vi "fFPGA Initialization.vi"(4 "Testpulse Cluster":T4={"Master Pulser On/Off"=FALSE, "Testpulse Turnaround Time (samples)"=14, "Pulse Separation (samples)"=0, "Pulse duration (samples)"=0}, 5 "DAQ Info Cluster":T3={"Data Chunks per File"=1000, "Samples per Waveform"=95, "Pretrigger Samples"=15, "circular buffer length (samples)"=1000, "Waveforms per Data Chunk"=5000} {"Waveforms per Data Chunk" format="%.2p"}, 6 "Channel Cluster":T2={"det_type"=[], "Serial numbers"=[], "Sources"=[], "Trigger level"=[4000, 4000, 4000, 4000, 4000, 4000, 4000, 4000], "Data Record On/Off"=[], "Number of Channels"=8}, 7 "General Cluster":cluster{"Location":i16} {"Location" items=["Purdue", "NIKHEF", "Zurich", "???"]}, 8 "error in":errorcluster, 11 "FPGA VI Reference In":T1) -> (0 "error out":errorcluster, 3 "FPGA VI Reference Out":T1)   [LabVIEW 2012]
uses:
  FPGA Bitfiles/ModuFPGAtype.ctl
  <vilib>/FPGAPlugInAG/PXI-7951R/niLvFpga_Reset_PXI-7951R.vi
  <vilib>/Utility/error.llb/Error Cluster From Error Code.vi
  <vilib>/LabVIEW Targets/FPGA/FlexRIO/CustomFPGAMethods/79XXR_Method_IOModuleStatusImpl.vi
  <vilib>/FPGAPlugInAG/PXI-7951R/niLvFpga_Run_PXI-7951R.vi
  <vilib>/rvi/errors/niLvFpgaAdjustHostInterfaceError.vi
  Program Files (x86)/National Instruments/LabVIEW 2012/Targets/NI/FPGA/StockFPGA_IntfPrivate/ScriptTemplates/StockFPGA_PlugInRead32.vi
  <vilib>/rvi/interface/nirviMethod/nirviMethod.xnode
  FPGA Bitfiles/ModuDAQ_FPGATarget_ModuFPGAdark_Chz-m0P+4co.lvbitx
  <vilib>/rvi/interface/nirviReadWriteControl/nirviReadWriteControl.xnode
  <vilib>/rvi/errors/niLvFpgaMergeErrorWithErrorCode.vi
  NiFpgaLv.dll
  <vilib>/FPGAPlugInAG/PXI-7951R/niLvFpga_Read32_PXI-7951R.vi
  <vilib>/rvi/interface/nirviReadWriteControl/niFpgaRWControlAccessTimeoutTemplate.vi
  <vilib>/FPGAPlugInAG/PXI-7951R/niLvFpga_ConfigureFifo_PXI-7951R.vi
  <vilib>/FPGAPlugInAG/PXI-7951R/niLvFpga_StartFifo_PXI-7951R.vi
panel:
  # "Channel 0"
  # "Channel 1"
  # "Channel 2"
  # "Channel 3"
  # "Channel 4"
  # "Channel 5"
  # "Channel 6"
  # "Channel 7"
  # "Waveform/Data Chunk information"
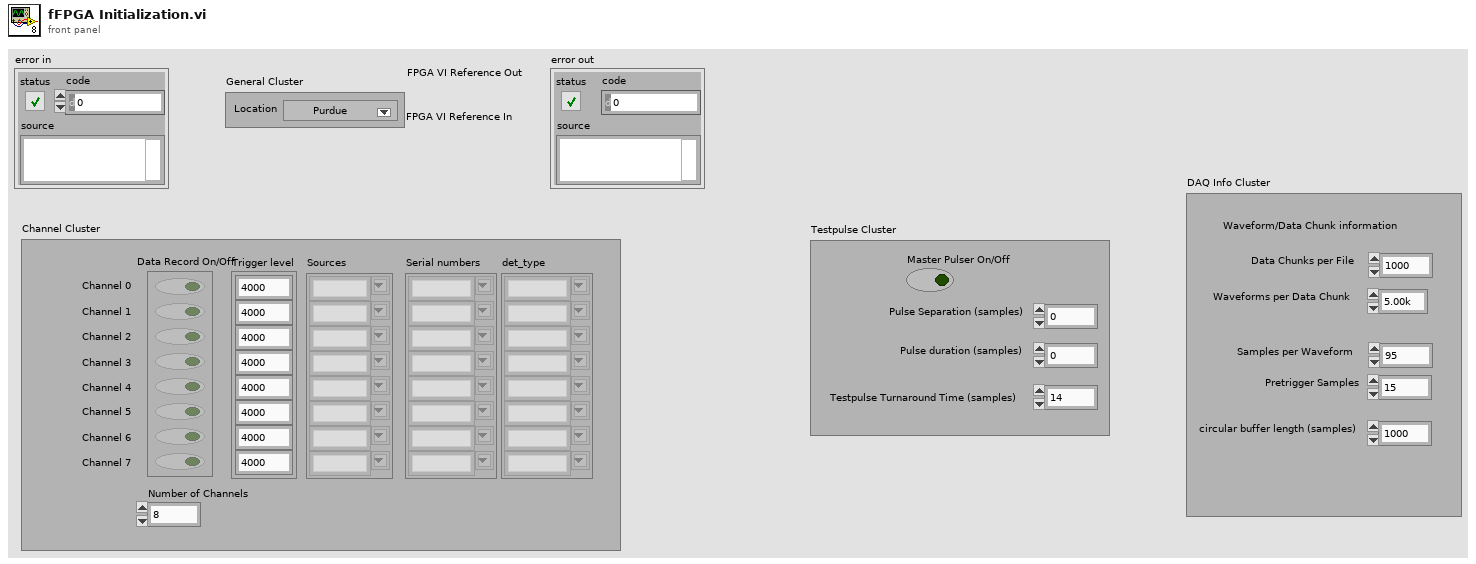
[diagram p1: front panel]
types:
  T1 = typedef "ModuFPGAtype.ctl" = refnum<k20>
  T2 = cluster{"det_type":string[], "Serial numbers":string[], "Sources":string[], "Trigger level":i16[], "Data Record On/Off":bool[], "Number of Channels":u8}
  T3 = cluster{"Data Chunks per File":u32, "Samples per Waveform":u32, "Pretrigger Samples":u32, "circular buffer length (samples)":u32, "Waveforms per Data Chunk":u32}
  T4 = cluster{"Master Pulser On/Off":bool, "Testpulse Turnaround Time (samples)":u32, "Pulse Separation (samples)":u32, "Pulse duration (samples)":u32}
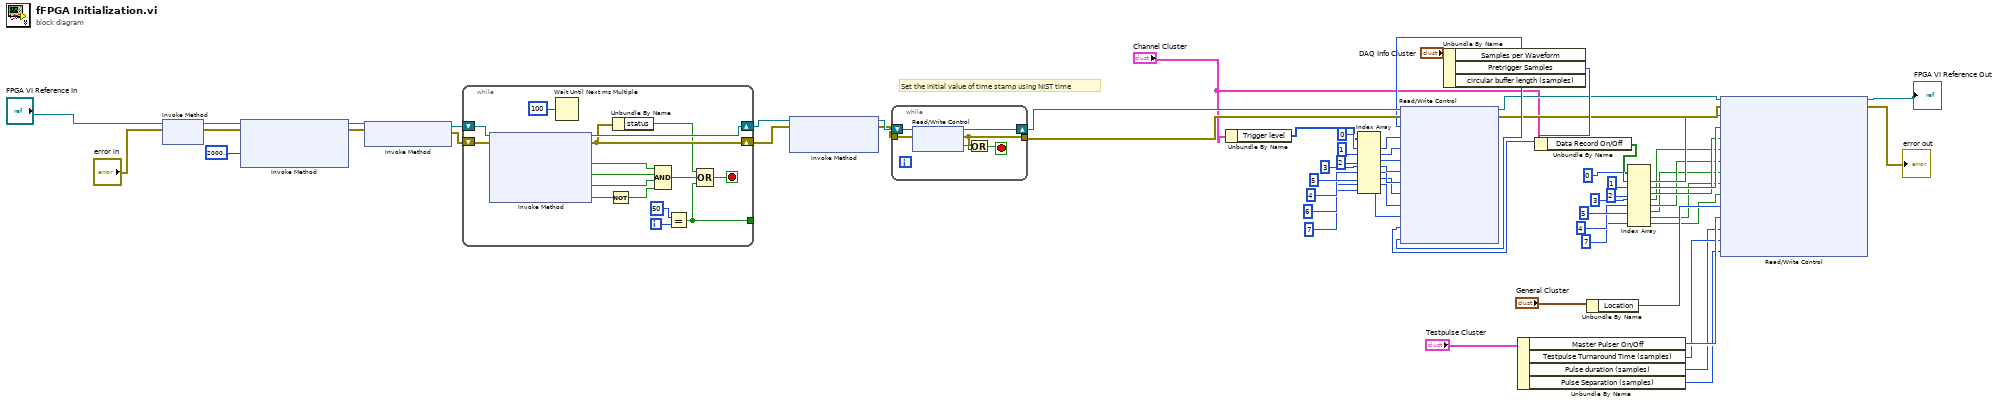
[diagram p0: block diagram]
diagram:
  # "Set the initial value of time stamp using NIST time"
  n1 = xnode "Invoke Method"("FPGA VI Reference In"="FPGA VI Reference In", "error in"="error in") -> ("FPGA VI Reference Out"=w49:T1, "error out"=w48:errorcluster)
  n2 = xnode "Invoke Method"("FPGA VI Reference In"=w49, "error in"=w48, "Requested Depth"=u32 20000000) -> ("FPGA VI Reference Out"=w52:T1, "error out"=w51:errorcluster)  [unwired: 1 out]
  n3 = xnode "Invoke Method"("FPGA VI Reference In"=w52, "error in"=w51) -> ("FPGA VI Reference Out"=w60:T1, "error out"=w59:errorcluster)
  n4 = while {
    shift-right: [w71] -> w53
    shift-left: w59 -> [w79]
    shift-right: [w78] -> w54
    shift-left: w60 -> [w80]
    tunnel: [w67] -> _
    i -> [w73]
    stop <- w68 stop-if-true
    n5 = xnode "Invoke Method"("FPGA VI Reference In"=w80, "error in"=w79) -> ("FPGA VI Reference Out"=w78:T1, "error out"=w71:errorcluster, "IO Module Present?"=w77:bool, "Power Enabled?"=w76:bool, "IO Enabled?"=w75:bool, "IO Module Mismatch?"=w66:bool)
    n6 = Wait Until Next ms Multiple(millisecond multiple=u32 100) -> ()  [unwired: 1 out]
    n7 = Not(x=w66) -> (.not. x?=w65:bool)
    n8 = Unbundle By Name(w71) -> ("status"=w70:bool)
    n9 = Compound Arithmetic op=AND(w77, w76, w75, w65) -> (w69:bool)
    n10 = Equal?(x=50, y=w73) -> (x = y?=w67:bool)
    n11 = Compound Arithmetic op=OR(w70, w69, w67) -> (w68:bool)
  }
  n12 = xnode "Invoke Method"("FPGA VI Reference In"=w54, "error in"=w53) -> ("FPGA VI Reference Out"=w63:T1, "error out"=w62:errorcluster)  [unwired: 1 in]
  n13 = while {
    tunnel: [w81] -> w46
    tunnel: w62 -> [w84]
    shift-right: [w86] -> w47
    shift-left: w63 -> [w85]
    stop <- w82 stop-if-true
    n14 = xnode "Read/Write Control"("FPGA VI Reference In"=w85, "error in"=w84) -> ("FPGA VI Reference Out"=w86:T1, "error out"=w81:errorcluster, "Init Done"=w83:bool)
    n15 = Or(x=w81, y=w83) -> (x .or. y?=w82:bool)
  }
  n16 = Unbundle By Name("Channel Cluster") -> ("Trigger level"=w58:i16[])
  n17 = Index Array(array=w58, index #1=0 ("index"), index #2=1 ("index"), index #3=2 ("index"), index #4=3 ("index"), index #5=4 ("index"), index #6=5 ("index"), index #7=6 ("index"), index #8=7 ("index")) -> (element #1=w45:i16, element #2=w26:i16, element #3=w25:i16, element #4=w24:i16, element #5=w23:i16, element #6=w22:i16, element #7=w21:i16, element #8=w20:i16)
  n18 = Unbundle By Name("DAQ Info Cluster") -> ("Samples per Waveform"=w42:u32, "Pretrigger Samples"=w43:u32, "circular buffer length (samples)"=w44:u32)
  n19 = xnode "Read/Write Control"("FPGA VI Reference In"=w47, "error in"=w46, "Record Size only data"=w42, "Trigger 0"=w45, "Trigger 1"=w26, "Trigger 2"=w25, "Trigger 3"=w24, "Trigger 4"=w23, "Trigger 5"=w22, "Trigger 6"=w21, "Trigger 7"=w20, "# of pretrigger"=w43, "circular buffer length"=w44) -> ("FPGA VI Reference Out"=w41:T1, "error out"=w39:errorcluster)
  n20 = Unbundle By Name("Testpulse Cluster") -> ("Master Pulser On/Off"=w37:bool, "Testpulse Turnaround Time (samples)"=w36:u32, "Pulse duration (samples)"=w35:u32, "Pulse Separation (samples)"=w3:u32)
  n21 = Unbundle By Name("Channel Cluster") -> ("Data Record On/Off"=w12:bool[])
  n22 = Unbundle By Name("General Cluster") -> ("Location"=w38:i16)
  n23 = Index Array(array=w12, index #1=0 ("index"), index #2=1 ("index"), index #3=2 ("index"), index #4=3 ("index"), index #5=4 ("index"), index #6=5 ("index"), index #8=7 ("index")) -> (element #1=w11:bool, element #2=w10:bool, element #3=w9:bool, element #4=w8:bool, element #5=w7:bool, element #6=w6:bool, element #7=w5:bool, element #8=w4:bool)  [unwired: 1 in]
  n24 = xnode "Read/Write Control"("FPGA VI Reference In"=w41, "error in"=w39, "channel 0 on/off"=w11, "channel 1 on/off"=w10, "channel 2 on/off"=w9, "channel 3 on/off"=w8, "channel 4 on/off"=w7, "channel 5 on/off"=w6, "channel 6 on/off"=w5, "channel 7 on/off"=w4, "location"=w38, "Testpulser On/Off"=w37, "Testpulse duration (20 ns ticks)"=w35, "Testpulse Time Delay (20 ns ticks)"=w36, "Testpulse Separation (20 ns ticks)"=w3) -> ("FPGA VI Reference Out"=→"FPGA VI Reference Out":T1, "error out"=→"error out":errorcluster)
